vi "Periodic Tasks.vi"(8 "error in":errorcluster) -> ()   [LabVIEW 2015]
doc: "This VI runs in parallel to other tasks. It can contain as many user-defined periodic loops as you need. These can carry out PID or other sorts of timed response."
uses:
  <vilib>/Rock Robotics/WPI/Solenoid/WPI_SolenoidValue.ctl
  Robot Global Data.vi
  <vilib>/Rock Robotics/WPI/Solenoid/WPI_SolenoidSetEnum.vi
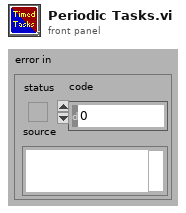
[diagram p1: front panel]
types:
  T1 = typedef "WPI_MotorControlDeviceRef.ctl" = cluster{"DeviceStatus":errorcluster, "Type":T2, "PWM":cluster{"PWM Channel":T3, "DeadBand":T4}, "CAN":cluster{"Device Number":u8, "Control Mode":T5, "Semaphore":T6, "Max Vout":dbl, "TalonSRX Control Mode":T7}, "Invert":bool}
  T2 = typedef "WPI_MotorControlType.ctl" = enum16{"PWM", "CAN", "CANTalonSRX"}
  T3 = typedef "FPGA_DIOPWMChannel.ctl" = enum8{"PWM 0", "PWM 1", "PWM 2", "PWM 3", "PWM 4", "PWM 5", "PWM 6", "PWM 7", "PWM 8", "PWM 9", "PWM MXP 0", "PWM MXP 1", "PWM MXP 2", "PWM MXP 3", "PWM MXP 4", "PWM MXP 5", "PWM MXP 6", "PWM MXP 7", "PWM MXP 8", "PWM MXP 9", "Invalid"}
  T4 = typedef "WPI_PWMDeadband.ctl" = cluster{"Name":string, "maxPositivePwm":i32, "minPositivePwm":i32, "centerPwm":i32, "maxNegativePwm":i32, "minNegativePwm":i32, "angularRange":u16}
  T5 = typedef "WPI_CANJaguar_ControlMode.ctl" = enum8{"Percent VBus", "Current", "Speed", "Position", "Voltage"}
  T6 = typedef "Semaphore RefNum" = refnum<k1>
  T7 = typedef "WPI_CANTalonSRX_APIControlMode.ctl" = enum8{"Percent VBus", "Speed", "Position", "Slave", "Unchanged / Invalid", "Voltage Compensation", "Current", "Motion Profile"}
  T8 = typedef "WPI_SolenoidDevRef.ctl" = cluster{"DevStatus":errorcluster, "Pneumatics Control Module":u8, "Forward Solenoid Channel":T9, "Reverse Solenoid Channel":T9}
  T9 = typedef "WPI_SolenoidChannel.ctl" = enum8{"Solenoid 0", "Solenoid 1", "Solenoid 2", "Solenoid 3", "Solenoid 4", "Solenoid 5", "Solenoid 6", "Solenoid 7", "Invalid"}
  T10 = typedef "WPI_SolenoidValue.ctl" = enum16{"Off", "On", "Forward", "Reverse"}
  T11 = cluster{"Joystick":cluster{"Intake motor axis":dbl, "Intake actuator axis":dbl, "Shifter button":bool}, "Cluster of sensors":cluster{"Sensor 1 input 2":u8, "Sensor 1 input 3":u8, "Sensor 1 input":u8, "Sensor 1 input 4":u8}}
  T12 = cluster{"Intake motor axis":dbl, "Intake actuator axis":dbl, "Shifter button":bool}
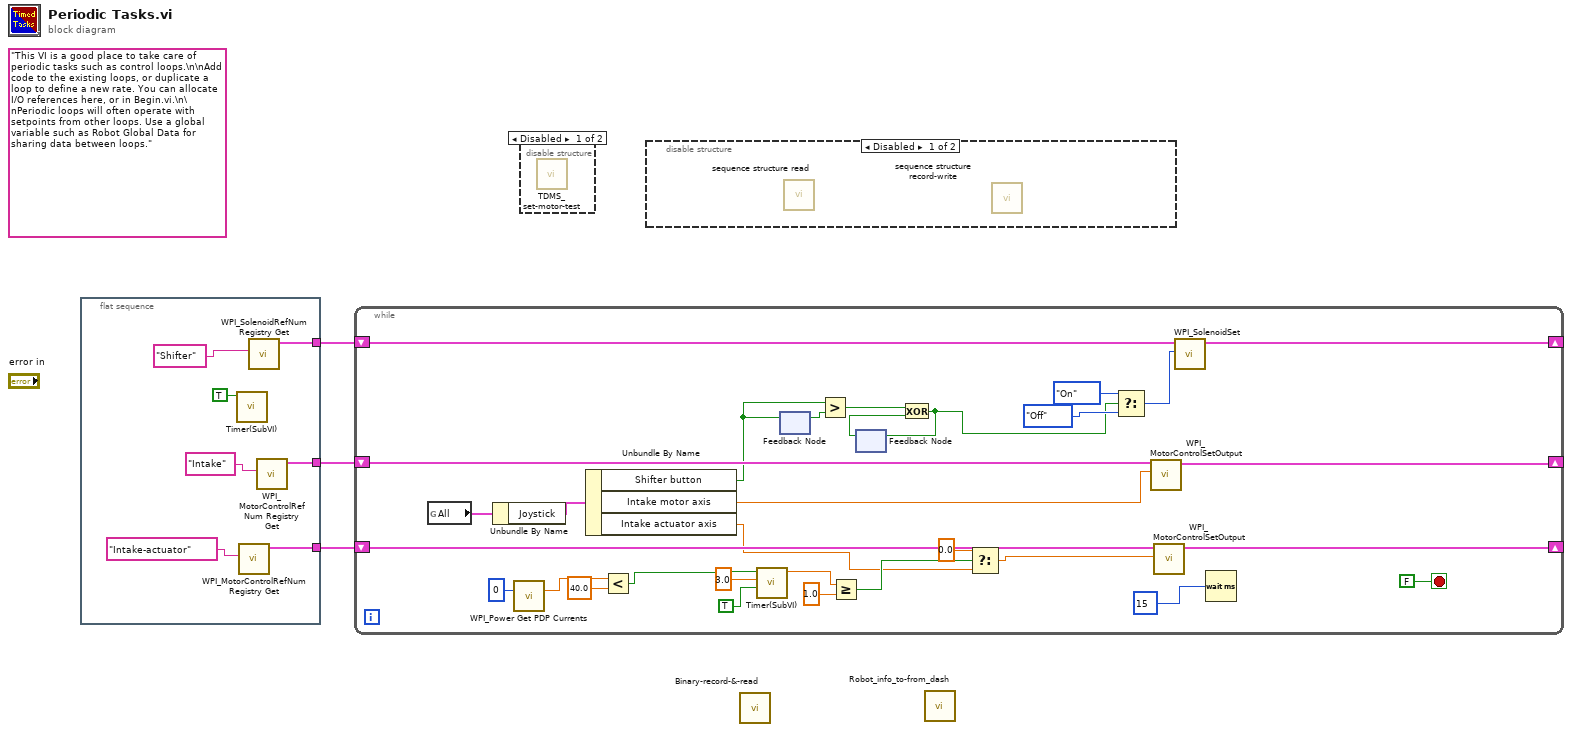
[diagram p0: block diagram]
diagram:
  (unwired) "This VI is a good place to take care of periodic tasks such as control loops.\n\nAdd code to the existing loops, or duplicate a loop to define a new rate. You can allocate I/O references here, or in Begin.vi.\n\nPeriodic loops will often operate with setpoints from other loops. Use a global variable such as Robot Global Data for sharing data between loops."
  n1 = flat-sequence {
    tunnel: [w9] -> w3
    tunnel: [w7] -> w2
    tunnel: [w5] -> w1
    frame #0 {
      n2 = call "Timer(SubVI).vi"("Reset?"=TRUE) -> ()  [unwired: 9 in, 2 out]
      n3 = call <vilib>:"WPI_MotorControlRefNum Registry Get.vi"("refnum name"="Intake-actuator") -> ("MotorControlDevRef"=w9:T1)  [unwired: 9 in, 1 out]
      n4 = call <vilib>:"WPI_SolenoidRefNum Registry Get.vi"("refnum name"="Shifter") -> ("SolenoidDevRef"=w5:T8)  [unwired: 9 in, 1 out]
      n5 = call <vilib>:"WPI_MotorControlRefNum Registry Get.vi"("refnum name"="Intake") -> ("MotorControlDevRef"=w7:T1)  [unwired: 9 in, 1 out]
    }
  }
  n6 = while {
    shift-right: [w37] -> _
    shift-left: w3 -> [w38]
    shift-right: [w36] -> _
    shift-left: w2 -> [w35]
    shift-right: [w31] -> _
    shift-left: w1 -> [w32]
    stop <- FALSE stop-if-true
    n7 = global read "Robot Global Data.vi" "All"() -> (w40:T11)
    n8 = Unbundle By Name(w40) -> ("Joystick"=w39:T12)
    n9 = call <vilib>:"WPI_Power Get PDP Currents.vi"("PDP Channel"=0) -> ("current (A)"=w13:dbl)  [unwired: 12 in, 2 out]
    n10 = Unbundle By Name(w39) -> ("Shifter button"=w23:bool, "Intake motor axis"=w34:dbl, "Intake actuator axis"=w16:dbl)
    n11 = Less?(x=w13, y=40.0) -> (x < y?=w11:bool)
    n12 = call "Timer(SubVI).vi"("Reset after time reached?"=TRUE, "Time to count up to"=3.0, "Reset?"=w11) -> ("Current time"=w20:dbl)  [unwired: 7 in, 1 out]
    n13 = feedback-in #1(w23) -> ()
    n14 = feedback #1() -> (w27:bool)  [unwired: 1 in]
    n15 = Greater?(x=w23, y=w27) -> (0:w26:bool)
    n16 = Greater Or Equal?(x=w20, y=1.0) -> (x >= y?=w17:bool)
    n17 = feedback #2() -> (w25:bool)  [unwired: 1 in]
    n18 = Exclusive Or(1:w25, 2:w26) -> (0:w24:bool)
    n19 = feedback-in #2(w24) -> ()
    n20 = Select(t=0.0, s=w17, f=w16) -> (s? t:f=w18:dbl)
    n21 = Select(t=WPI_SolenoidValue."On", s=w24, f=WPI_SolenoidValue."Off" ("Value")) -> (s? t:f=w29:T10)
    n22 = call <vilib>:"WPI_MotorControlSetOutput.vi"("Output"=w34, "MotorControlDevRef"=w35) -> ("MotorControlDevRef"=w36:T1)  [unwired: 7 in, 2 out]
    n23 = call <vilib>:"WPI_MotorControlSetOutput.vi"("Output"=w18, "MotorControlDevRef"=w38) -> ("MotorControlDevRef"=w37:T1)  [unwired: 7 in, 2 out]
    n24 = call-poly <vilib>:"WPI_SolenoidSet.vi"("Value"=w29, "SolenoidDevRef"=w32) -> ("SolenoidDevRef"=w31:T8)  [unwired: 8 in, 1 out]
    n25 = Wait (ms)(milliseconds to wait=u32 15) -> ()  [unwired: 1 out]
  }
  n26 = disable-structure shown="Disabled" {
    frame Disabled {
      n27 = call "TDMS_set-motor-test.vi"() -> ()  [unwired: 12 in]
    }
    frame Enabled {
    }
  }
  n28 = disable-structure shown="Disabled" {
    frame Disabled {
      n29 = call "sequence structure read.vi"() -> ()  [unwired: 12 in]
      n30 = call "sequence structure record-write.vi"() -> ()  [unwired: 12 in]
    }
    frame Enabled {
    }
  }
  n31 = call "Binary-record-&-read.vi"() -> ()  [unwired: 12 in]
  n32 = call "Robot_info_to-from_dash.vi"() -> ()  [unwired: 12 in]
